vi "send.vi"(0 "baud rate":u32=9600 caption="波特率", 1 "文件路径":path=path "C:/Users/Twsa/Desktop/3Dprinter_labview/gcode_exe/fileFinal.txt", 2 "端口":refnum<visa-resource-name>="COM4", 3 "数值":dbl=102400.0) -> ()   [LabVIEW 2018]
uses:
  <vilib>/Instr/_visa.llb/VISA Configure Serial Port (Instr).vi
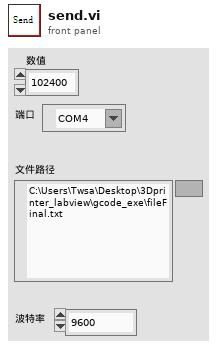
[diagram p1: front panel]
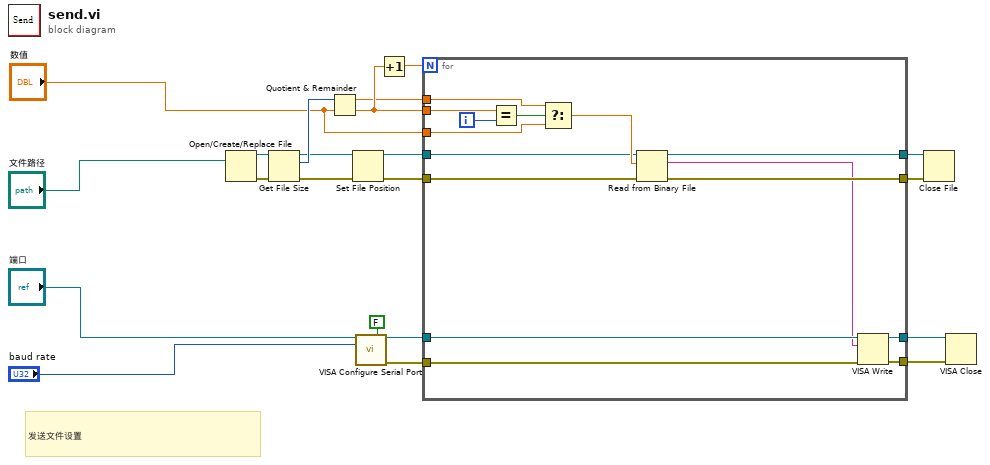
[diagram p0: block diagram]
diagram:
  # "发送文件设置"
  n1 = Open/Create/Replace File(file path (use dialog)="文件路径") -> (refnum out=w14:refnum<file>, error out=w15:errorcluster)  [unwired: 5 in, 1 out]
  n2 = Get File Size(file=w14, error in=w15) -> (refnum out=w8:refnum<file>, size (in bytes)=w13:i64, 0:w6:errorcluster)
  n3 = Quotient & Remainder(x=w13, y="数值") -> (x-y*floor(x/y)=w10:dbl, floor(x/y)=w12:dbl)
  n4 = Set File Position(refnum=w8, error in=w6) -> (refnum out=w7:refnum<file>, error out=w5:errorcluster)  [unwired: 2 in]
  n5 = call-poly "VISA Configure Serial Port"("VISA resource name"="端口", "Enable Termination\nChar (T)"=FALSE ("Enable Termination\nChar (T)"), "baud rate (9600)"="baud rate") -> ("VISA resource name out"=w21:refnum<visa-resource-name>, "error out"=w20:errorcluster)  [unwired: 11 in]
  n6 = Increment(x=w12) -> (x+1=w11:dbl)
  n7 = for {
    N: w11 -> [_]
    tunnel: w21 -> [w32]
    tunnel: w20 -> [w31]
    tunnel: [w36] -> w17
    tunnel: [w35] -> w16
    tunnel: w7 -> [w24]
    tunnel: w5 -> [w23]
    tunnel: [w34] -> w19
    tunnel: [w33] -> w18
    tunnel: "数值" -> [w27]
    tunnel: w12 -> [w30]
    tunnel: w10 -> [w28]
    i -> [w22]
    n8 = Equal?(x=w30, y=w22) -> (x = y?=w29:bool)
    n9 = Select(t=w28, s=w29, f=w27) -> (s? t:f=w26:dbl)
    n10 = Read from Binary File(8:w23, 10:w26, 11:w24) -> (0:w33:errorcluster, 2:w25:string, 3:w34:refnum<file>)  [unwired: 3 in, 1 out]
    n11 = VISA Write(VISA resource name=w32, write buffer=w25, error in (no error)=w31) -> (VISA resource name out=w36:refnum<visa-resource-name>, error out=w35:errorcluster)  [unwired: 1 out]
  }
  n12 = Close File(refnum=w19, error in=w18) -> ()  [unwired: 2 out]
  n13 = VISA Close(VISA resource name=w17, error in (no error)=w16) -> ()  [unwired: 1 out]
